vi "参数设置页.vi"() -> ()   [LabVIEW 2016, in "斯坦道总磷总氮.lvlib"]
uses:
  <vilib>/Plasmionique/MB Master/MB_Master/MB_Master.lvclass
  <vilib>/ptbypt/NI_PtbyPt.lvlib
panel:
  in  "简易流程路径":path=path "data/流程.xml"
  out "数据刷新时间":string
  in  "通讯连接":bool
  out "MB table":enum32{"Serial", "TCP"}(tab)
  in  "请选择串口:":refnum<visa-resource-name>
  in  "IP":string="127.0.0.1"
  in  "PORT":string="1001"
  in  "通信方式选择":enum16{"串口", "TCP"}(ring)
  in  "盐度自动补偿：":bool
  out "盐度补偿值":dbl caption="盐度补偿值："
  in  "刷新":bool
  in  "测量模式":T1(ring)
  in  "参数下拉列表":u16(ring) items=["总磷"=1, "总氮"=2]
  in  "量程下拉列表":enum16{"低量程", "高量程"}(ring)
  in  "测试流程路径":path=path "data/流程.xml"
  in  "标样核查量程模式":enum16{"高量程", "低量程", "自动"}(ring) caption="标样核查量程模式："
  in  "加标回收量程模式":enum16{"高量程", "低量程", "自动"}(ring) caption="加标回收量程模式："
  in  "跨度核查量程模式":enum16{"高量程", "低量程", "自动"}(ring) caption="跨度核查量程模式："
  in  "零点核查量程模式":enum16{"高量程", "低量程", "自动"}(ring) caption="零点核查量程模式："
  in  "水样测试量程模式":enum16{"高量程", "低量程", "自动"}(ring) caption="水样测试量程模式："
  out "稀释度":dbl caption="稀释度："
  out "阈值（高->低）":dbl caption="阈值（高->低）："
  out "阈值（低->高）":dbl caption="阈值（低->高）："
  out "量程下限":dbl caption="量程下限："
  out "量程上限":dbl caption="量程上限："
  out "检出限":dbl caption="检出限："
  out "曲线截距":dbl caption="曲线截距：" format="%#.6f"
  out "曲线斜率":dbl caption="曲线斜率：" format="%#.6f"
  out "二次多项式系数":dbl caption="二次多项式系数：" format="%#.6f"
  out "消解时长":dbl caption="消解时长："
  out "消解温度":dbl caption="消解温度："
  out "测量精度":u16 caption="测量精度："
  in  "标样核查标液浓度":dbl caption="标样核查标液浓度："
  in  "跨度核查标液浓度":dbl caption="跨度核查标液浓度："
  in  "零点核查标液浓度":dbl caption="零点核查标液浓度："
  in  "跨度值":dbl caption="跨度值："
  # "ppt"
  # "mg/L"
  # "mg/L"
  # "mg/L"
  # "mg/L"
  # "mg/L"
  # "min"
  # "℃"
  # "mg/L"
  # "mg/L"
  # "mg/L"
  # "mg/L"
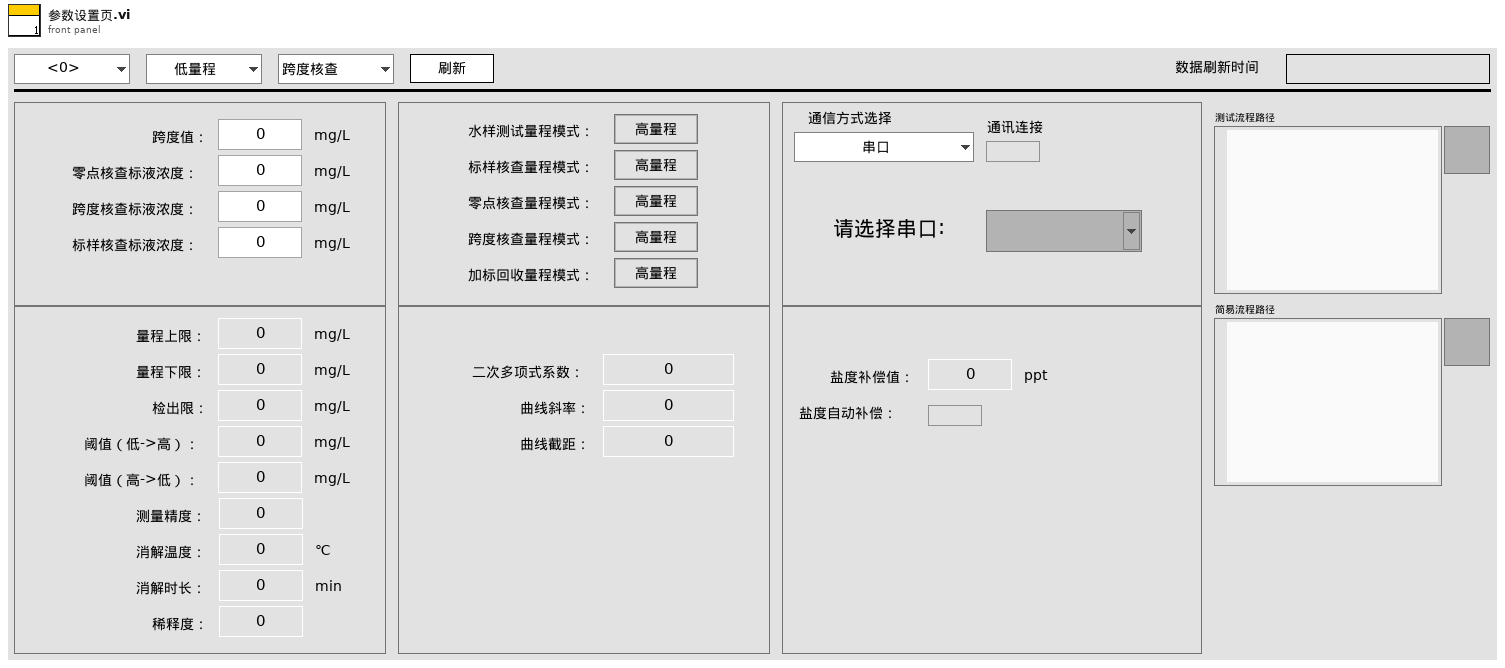
[diagram p1: front panel]
types:
  T1 = enum16{"跨度核查", "水样测量", "零点核查", "标样核查", "加标回收", "快捷测试", "空白校准", "标样校准"}
  T2 = enum8{"Enabled", "Disabled", "Disabled and Grayed Out"}
  T3 = typedef "LVStringsAndValuesArrayTypeDef_U16.ctl" = cluster{"String":string, "Value":u16}[]
  T4 = cluster{"标液浓度1":dbl, "测量吸光度1":dbl, "样品1启用":bool, "标液浓度2":dbl, "测量吸光度2":dbl, "样品2启用":bool, "标液浓度3":dbl, "测量吸光度3":dbl, "样品3启用":bool, "标液浓度4":dbl, "测量吸光度4":dbl, "样品4启用":bool, "标液浓度5":dbl, "测量吸光度5":dbl, "样品5启用":bool, "模型":enum32{"线性", "多项式"}, "精度":dbl, "XY图":cluster{"X Values":dbl[], "Y Values":dbl[]}[], "拟合公式":string, "r^2":dbl, "标样一校准时间":timestamp, "标样二校准时间":timestamp, "标样三校准时间":timestamp, "标样四校准时间":timestamp, "标样五校准时间":timestamp, "二次方程":cluster{"c":dbl, "x":dbl, "x^2":dbl}, "标定时间":timestamp}
  T5 = cluster{"系统时间":timestamp, "工作状态":u16, "测量模式":enum16{"待机", "连续模式", "周期模式", "定点模式", "受控模式", "手动模式"}, "告警代码":u16, "故障代码":u16, "日志代码":u16, "软件版本":u16, "F0":sgl, "F1":sgl, "F2":sgl, "F3":sgl, "T":sgl, "H":sgl, "id":u16, "flowid":u16, "量程":u16, "总磷控温温度1":sgl, "营养盐控温温度2":sgl, "ADC":sgl}
  T6 = cluster{"测量精度":u16, "检出限":dbl, "上限":dbl, "下限":dbl, "阈值（低->高）":dbl, "阈值（高->低）":dbl, "稀释度":dbl}
  T7 = cluster{"泵类型":u8, "进样速度":u32, "出样速度":u32, "泵阀量":u8, "光谱仪类型":u8, "光谱采样次数":u8, "氙灯次数":u8, "B":u16, "C":u16, "D":u16, "E":u16, "B_COD":u16, "C_COD":u16, "D_COD":u16, "E_COD":u16, "G":u16, "M":u16, "N":u16, "氨氮注射泵控温下限":sgl, "氨氮注射泵控温上限":sgl, "总氮注射泵控温下限":sgl, "总氮注射泵控温上限":sgl, "消解温度下限":sgl, "消解温度上限":sgl, "加热10s限值":sgl, "高温高压阀开阀温度":sgl, "总氮x公式0":u8, "总氮x公式1":sgl, "总氮x公式2":sgl, "总磷浊度稀释系数":sgl, "总磷浊度补偿权重1":sgl, "总磷浊度补偿权重2":sgl, "盐度系数":sgl, "氨氮补偿系数1":sgl, "氨氮补偿系数2":sgl}
  T8 = cluster{"标液浓度1":dbl, "测量吸光度1":dbl, "样品1启用":bool, "标液浓度2":dbl, "测量吸光度2":dbl, "样品2启用":bool, "标液浓度3":dbl, "测量吸光度3":dbl, "样品3启用":bool, "标液浓度4":dbl, "测量吸光度4":dbl, "样品4启用":bool, "标液浓度5":dbl, "测量吸光度5":dbl, "样品5启用":bool, "模型":enum32{"线性", "多项式"}, "精度":dbl, "XY图":cluster{"X Values":dbl[], "Y Values":dbl[]}[], "拟合公式":string, "r^2":dbl, "标样一校准时间":timestamp, "标样二校准时间":timestamp, "标样三校准时间":timestamp, "标样四校准时间":timestamp, "标样五校准时间":timestamp, "二次方程":cluster{"c":dbl, "x":dbl, "x^2":dbl}, "标定时间":timestamp}[]
  T9 = typedef "斯坦道总磷总氮.lvlib/关键参数.ctl" = cluster{"测量量程":sgl, "测量检出限":sgl, "测量精度":sgl, "测量间隔":sgl, "消解温度":sgl, "消解时长":sgl, "三项式系数":sgl, "二次多项式系数":sgl, "曲线斜率":sgl, "曲线截距":sgl, "线性相关系数":sgl, "空白校准时间":timestamp, "标样校准时间":timestamp, "测量信号值":sgl, "稀释倍数":sgl, "空白标定系数":sgl, "量程系数":sgl}
  T10 = cluster{"水样测试量程模式":enum16{"高量程", "低量程", "自动"}, "零点核查量程模式":enum16{"高量程", "低量程", "自动"}, "跨度核查量程模式":enum16{"高量程", "低量程", "自动"}, "加标回收量程模式":enum16{"高量程", "低量程", "自动"}, "标样核查量程模式":enum16{"高量程", "低量程", "自动"}}
  T11 = cluster{"总磷跨度值":dbl, "总磷零点标准液浓度":dbl, "总磷跨度标准液浓度":dbl, "总磷标准液标准浓度":dbl, "总氮跨度值":dbl, "总氮零点标准液浓度":dbl, "总氮跨度标准液浓度":dbl, "总氮标准液标准浓度":dbl, "COD跨度值":dbl, "COD零点标准液浓度":dbl, "COD跨度标准液浓度":dbl, "COD标准液标准浓度":dbl, "氨氮跨度值":dbl, "氨氮零点标准液浓度":dbl, "氨氮跨度标准液浓度":dbl, "氨氮标准液标准浓度":dbl, "磷酸盐跨度值":dbl, "磷酸盐零点标准液浓度":dbl, "磷酸盐跨度标准液浓度":dbl, "磷酸盐标准液标准浓度":dbl, "硝氮跨度值":dbl, "硝氮零点标准液浓度":dbl, "硝氮跨度标准液浓度":dbl, "硝氮标准液标准浓度":dbl, "亚硝氮跨度值":dbl, "亚硝氮零点标准液浓度":dbl, "亚硝氮跨度标准液浓度":dbl, "亚硝氮标准液标准浓度":dbl, "硫化物跨度值":dbl, "硫化物零点标准液浓度":dbl, "硫化物跨度标准液浓度":dbl, "硫化物标准液标准浓度":dbl, "硅酸盐跨度值":dbl, "硅酸盐零点标准液浓度":dbl, "硅酸盐跨度标准液浓度":dbl, "硅酸盐标准液标准浓度":dbl}
  T12 = cluster{"水样测试量程模式":u16, "零点核查量程模式":u16, "跨度核查量程模式":u16, "加标回收量程模式":u16, "标样核查量程模式":u16}
  T13 = cluster{"水样测试量程模式":enum16{"H", "L", "AUTO"}, "空白核查量程模式":enum16{"H", "L", "AUTO"}, "跨度核查量程模式":enum16{"H", "L", "AUTO"}, "加标回收量程模式":enum16{"H", "L", "AUTO"}, "标样核查量程模式":enum16{"H", "L", "AUTO"}}
  T14 = cluster{"水样测试量程模式":u16, "空白核查量程模式":u16, "跨度核查量程模式":u16, "加标回收量程模式":u16, "标样核查量程模式":u16}
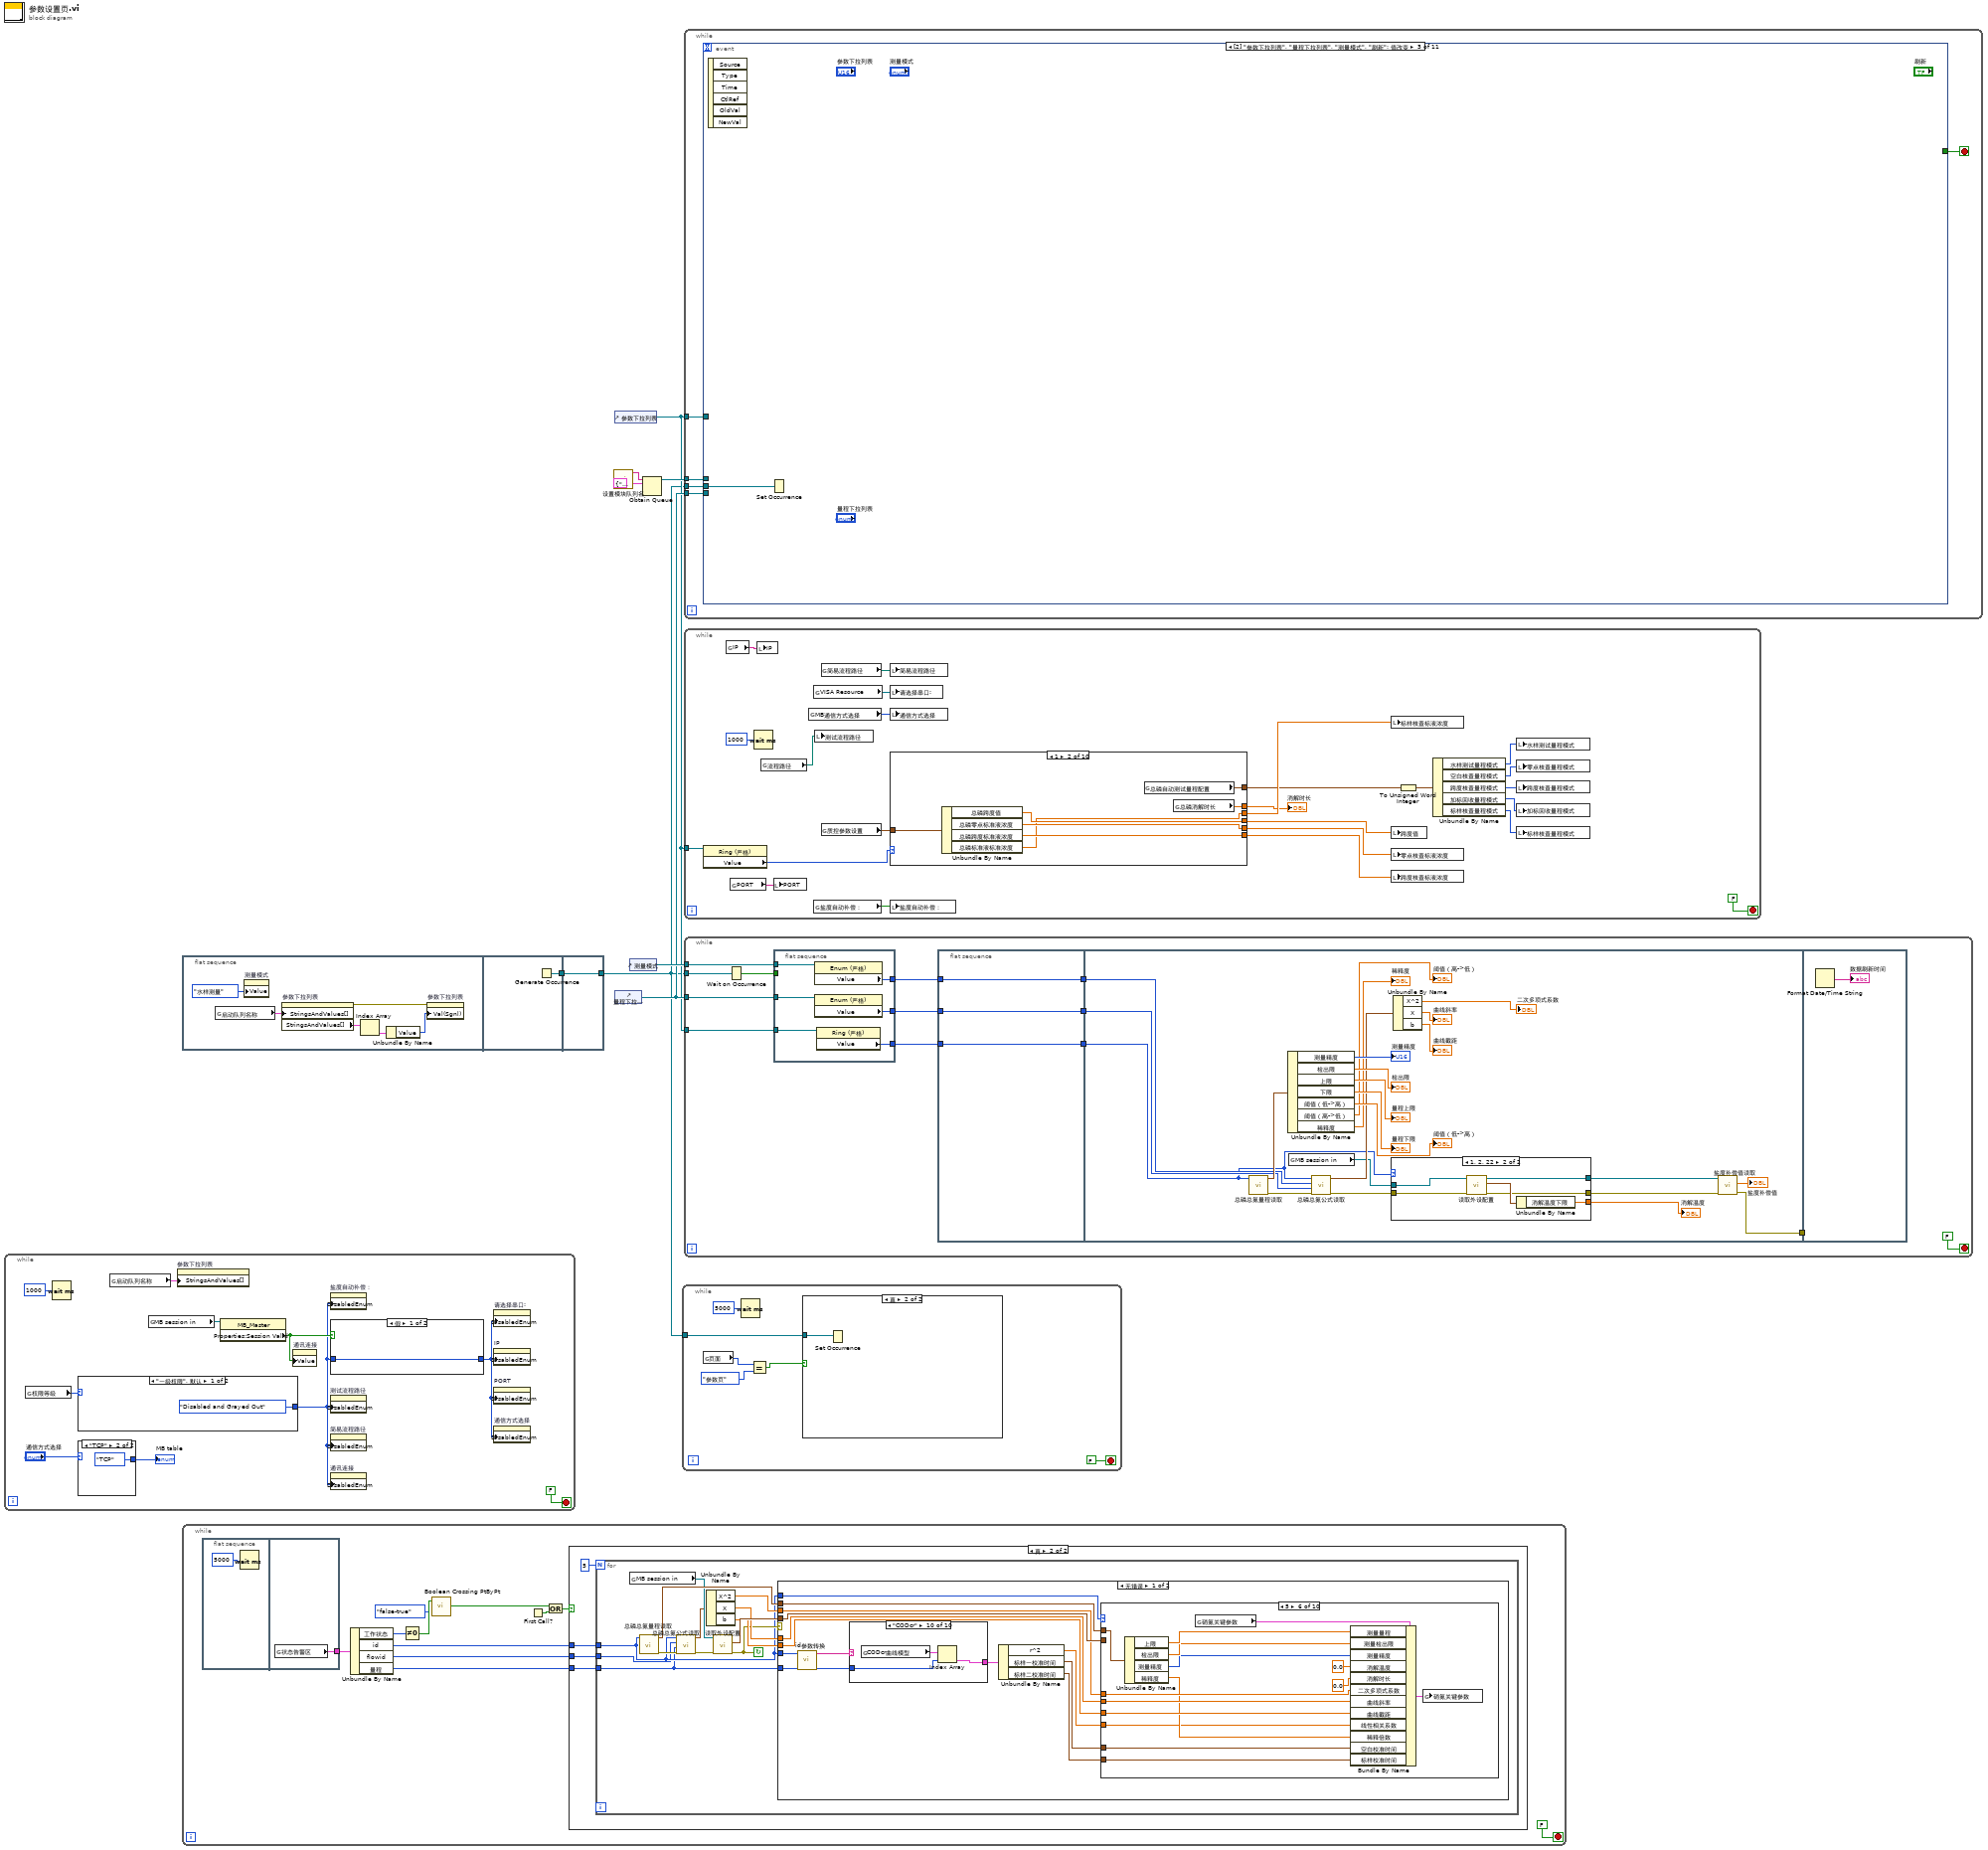
[diagram p0: block diagram]
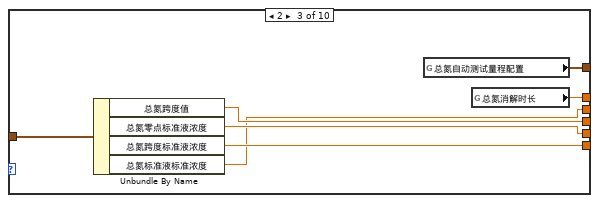
[diagram p4: hidden frame]
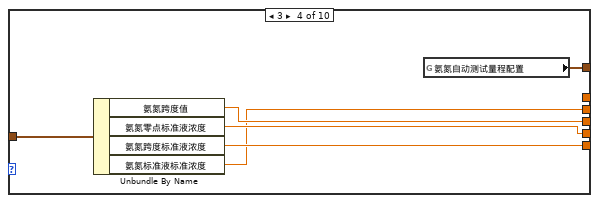
[diagram p5: hidden frame]
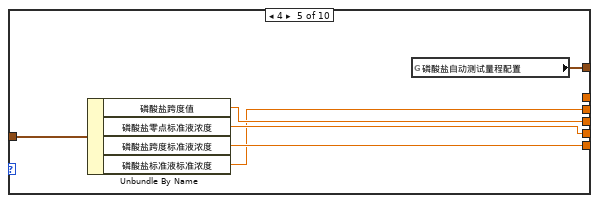
[diagram p6: hidden frame]
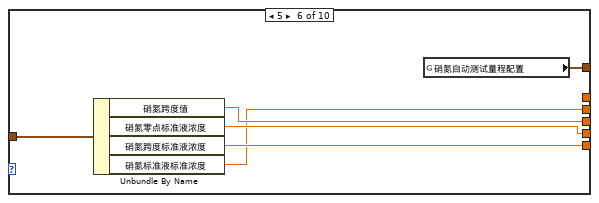
[diagram p7: hidden frame]
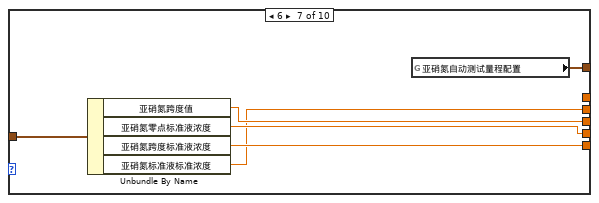
[diagram p8: hidden frame]
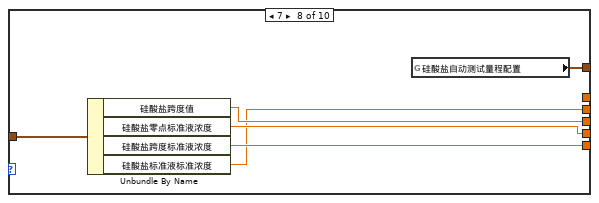
[diagram p9: hidden frame]
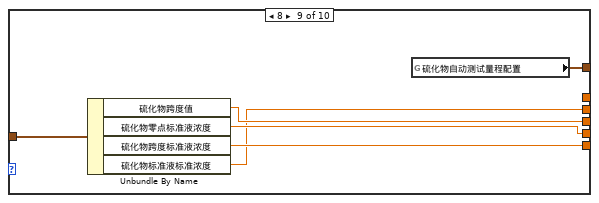
[diagram p10: hidden frame]
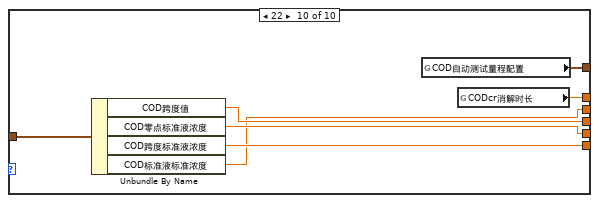
[diagram p11: hidden frame]
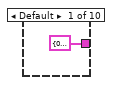
[diagram p13: hidden frame]
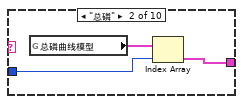
[diagram p14: hidden frame]
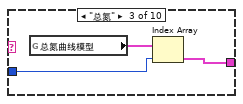
[diagram p15: hidden frame]
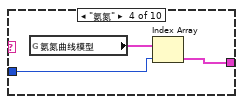
[diagram p16: hidden frame]
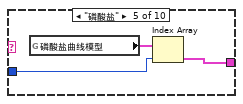
[diagram p17: hidden frame]
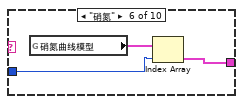
[diagram p18: hidden frame]
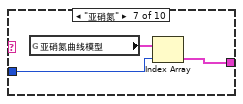
[diagram p19: hidden frame]
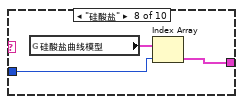
[diagram p20: hidden frame]
diagram:
  n1 = while {
    stop <- FALSE stop-if-true
    n2 = global read "VAR总磷总氮全局变量.vi" "权限等级"() -> (w11:enum16{"一级权限", "二级权限", "三级权限", "超级权限"})
    n3 = Wait (ms)(milliseconds to wait=u32 1000 ("等待时间（毫秒）")) -> ()  [unwired: 1 out]
    n4 = case shown="\"一级权限\", 默认" w11 {
      tunnel: [T2."Disabled and Grayed Out" ("禁用") T2."Enabled" ("禁用")] -> w10
      frame "一级权限", Default {
      }
      frame "二级权限".."超级权限" {
      }
    }
    n5 = case shown="\"TCP\"" "通信方式选择" {
      tunnel: [enum32{"Serial", "TCP"}."Serial" ("MB table") enum32{"Serial", "TCP"}."TCP" ("MB table")] -> w13
      frame "串口", Default {
      }
      frame "TCP" {
      }
    }
    "MB table" <- w13
    n6 = global read "总磷总氮断电保存全局变量.vi" "启动队列名称"() -> (w9:cluster{"String":string, "Value":u16}[])
    n7 = global read "VAR总磷总氮全局变量.vi" "MB session in"() -> (w17:refnum<class "MB_Master.lvclass">)
    n8 = property on="参数下拉列表" class="Ring (严格)"("StringsAndValues[]"=w9) -> ()  [unwired: 2 in, 2 out]
    n9 = property class="MB_Master"(reference=w17) -> ("Properties:Session Valid"=w15:bool)  [unwired: 1 in, 2 out]
    n10 = property on="通讯连接" class="Bool (严格)"("Value"=w15) -> ()  [unwired: 2 in, 2 out]
    n11 = property on="盐度自动补偿：" class="Bool (严格)"("DisabledEnum"=w10) -> ()  [unwired: 2 in, 2 out]
    n12 = case shown="假" w15 {
      tunnel: [w23 T2."Disabled and Grayed Out" ("禁用")] -> w14
      tunnel: w10 -> [w23 _]
      frame False {
      }
      frame True {
      }
    }
    n13 = property on="测试流程路径" class="Path"("DisabledEnum"=w10) -> ()  [unwired: 2 in, 2 out]
    n14 = property on="简易流程路径" class="Path"("DisabledEnum"=w10) -> ()  [unwired: 2 in, 2 out]
    n15 = property on="通讯连接" class="Bool (严格)"("DisabledEnum"=w10) -> ()  [unwired: 2 in, 2 out]
    n16 = property on="请选择串口:" class="VISAName"("DisabledEnum"=w14) -> ()  [unwired: 2 in, 2 out]
    n17 = property on="IP" class="Str"("DisabledEnum"=w14) -> ()  [unwired: 2 in, 2 out]
    n18 = property on="PORT" class="Str"("DisabledEnum"=w14) -> ()  [unwired: 2 in, 2 out]
    n19 = property on="通信方式选择" class="Enum (严格)"("DisabledEnum"=w14) -> ()  [unwired: 2 in, 2 out]
  }
  n20 = flat-sequence {
    tunnel: [w31] -> w8
    tunnel: [w32] -> w1
    tunnel: w8 -> [w32]
    frame #0 {
      n21 = global read "总磷总氮断电保存全局变量.vi" "启动队列名称"() -> (w26:cluster{"String":string, "Value":u16}[])
      n22 = property on="测量模式" class="Enum (严格)"("Value"=T1."水样测量" ("测量模式")) -> ()  [unwired: 2 in, 2 out]
      n23 = property on="参数下拉列表" class="Ring (严格)"("StringsAndValues[]"=w26) -> (error out=w29:errorcluster, "StringsAndValues[]"=w27:T3)  [unwired: 2 in, 1 out]
      n24 = Index Array(array=w27) -> (element=w28:cluster{"String":string, "Value":u16})  [unwired: 1 in]
      n25 = Unbundle By Name(w28) -> ("Value"=w30:u16)
      n26 = property on="参数下拉列表" class="Ring (严格)"(error in=w29, "Val(Sgnl)"=w30) -> ()  [unwired: 1 in, 2 out]
    }
    frame #1 {
      n27 = Generate Occurrence() -> (w31:refnum<k4>)
    }
    frame #2 {
    }
  }
  n28 = while {
    stop <- FALSE stop-if-true
    n29 = flat-sequence {
      tunnel: [w45] -> w43
      frame #0 {
        n30 = Wait (ms)(milliseconds to wait=u32 5000 ("等待时间（毫秒）")) -> ()  [unwired: 1 out]
      }
      frame #1 {
        n31 = global read "VAR总磷总氮全局变量.vi" "状态告警区"() -> (w45:T5)
      }
    }
    n32 = Unbundle By Name(w43) -> ("工作状态"=w39:u16, "id"=w40:u16, "flowid"=w41:u16, "量程"=w42:u16)
    n33 = Not Equal To 0?(x=w39) -> (x != 0?=w38:bool)
    n34 = call <vilib>:"Boolean Crossing PtByPt.vi"("direction"=enum16{"either", "false-true", "true-false"}."false-true", "input"=w38) -> ("crossing"=w36:bool)  [unwired: 1 in]
    n35 = First Call?() -> (First Call?: T/F=w33:bool)
    n36 = Or(x=w36, y=w33) -> (x .or. y?=w34:bool)
    n37 = case shown="真" w34 {
      tunnel: w42 -> [_ w49]
      tunnel: w41 -> [_ w48]
      tunnel: w40 -> [_ w47]
      frame False {
      }
      frame True {
        n38 = for {
          N: 5 -> [_]
          tunnel: w49 -> [w51]
          tunnel: w48 -> [w50]
          tunnel: w47 -> [w52]
          stop <- w53 continue-if-true
          n39 = global read "VAR总磷总氮全局变量.vi" "MB session in"() -> (w61:refnum<class "MB_Master.lvclass">)
          n40 = call "总磷总氮量程读取.vi"("测量参数"=w52) -> ("error out"=w55:errorcluster, "量程参数读取"=w62:T6)  [unwired: 9 in]
          n41 = call "总磷总氮公式读取.vi"("error in (no error)"=w55, "量程"=w51, "测量模式"=w50, "测量参数"=w52) -> ("error out"=w54:errorcluster, "公式"=w59:cluster{"X^2":dbl, "X":dbl, "b":dbl})  [unwired: 6 in]
          n42 = Unbundle By Name(w59) -> ("X^2"=w58:dbl, "X"=w57:dbl, "b"=w56:dbl)
          n43 = call "读取外设配置.vi"("error in (no error)"=w54, "MB session in"=w61) -> ("error out"=w53:errorcluster, "外设配置"=w60:T7)  [unwired: 7 in, 1 out]
          n44 = case shown="无错误" w53 {
            tunnel: w62 -> [w75 _]
            tunnel: w60 -> [w74 _]
            tunnel: w58 -> [w73 _]
            tunnel: w57 -> [w72 _]
            tunnel: w56 -> [w71 _]
            tunnel: w52 -> [w70 _]
            tunnel: w52 -> [w67 _]
            tunnel: w51 -> [w63 _]
            frame No Error {
              n45 = call "id参数转换.vi"("id"=w67) -> ("table输出"=w69:string)  [unwired: 9 in, 1 out]
              n46 = case shown="\"CODcr\"" w69 {
                tunnel: w63 -> [_ w77 w80 w83 w86 w89 w92 w95 w98 w101]
                tunnel: [T4 {"标液浓度1"=0.0, "测量吸光度1"=0.0, "样品1启用"=FALSE, "标液浓度2"=0.0, "测量吸光度2"=0.0, "样品2启用"=FALSE, "标液浓度3"=0.0, "测量吸光度3"=0.0, "样品3启用"=FALSE, "标液浓度4"=0.0, "测量吸光度4"=0.0, "样品4启用"=FALSE, "标液浓度5"=0.0, "测量吸光度5"=0.0, "样品5启用"=FALSE, "模型"=enum."线性", "精度"=0.0, "XY图"=[], "拟合公式"="", "r^2"=0.0, "标样一校准时间"=timestamp(0 s since 1904-01-01), "标样二校准时间"=timestamp(0 s since 1904-01-01), "标样三校准时间"=timestamp(0 s since 1904-01-01), "标样四校准时间"=timestamp(0 s since 1904-01-01), "标样五校准时间"=timestamp(0 s since 1904-01-01), "二次方程"={"c"=0.0, "x"=0.0, "x^2"=0.0}, "标定时间"=timestamp(0 s since 1904-01-01)} ("总磷曲线模型") w78 w81 w84 w87 w90 w93 w96 w99 w102] -> w68
                frame Default {
                }
                frame "总磷" {
                  n47 = global read "校准数据全局变量.vi" "总磷曲线模型"() -> (w79:T8)
                  n48 = Index Array(array=w79, index=w77) -> (element=w78:T4)
                }
                frame "总氮" {
                  n49 = global read "校准数据全局变量.vi" "总氮曲线模型"() -> (w82:T8)
                  n50 = Index Array(array=w82, index=w80) -> (element=w81:T4)
                }
                frame "氨氮" {
                  n51 = global read "校准数据全局变量.vi" "氨氮曲线模型"() -> (w85:T8)
                  n52 = Index Array(array=w85, index=w83) -> (element=w84:T4)
                }
                frame "磷酸盐" {
                  n53 = global read "校准数据全局变量.vi" "磷酸盐曲线模型"() -> (w88:T8)
                  n54 = Index Array(array=w88, index=w86) -> (element=w87:T4)
                }
                frame "硝氮" {
                  n55 = global read "校准数据全局变量.vi" "硝氮曲线模型"() -> (w91:T8)
                  n56 = Index Array(array=w91, index=w89) -> (element=w90:T4)
                }
                frame "亚硝氮" {
                  n57 = global read "校准数据全局变量.vi" "亚硝氮曲线模型"() -> (w94:T8)
                  n58 = Index Array(array=w94, index=w92) -> (element=w93:T4)
                }
                frame "硅酸盐" {
                  n59 = global read "校准数据全局变量.vi" "硅酸盐曲线模型"() -> (w97:T8)
                  n60 = Index Array(array=w97, index=w95) -> (element=w96:T4)
                }
                frame "硫化物" {
                  n61 = global read "校准数据全局变量.vi" "硫化物曲线模型"() -> (w100:T8)
                  n62 = Index Array(array=w100, index=w98) -> (element=w99:T4)
                }
                frame "CODcr" {
                  n63 = global read "校准数据全局变量.vi" "CODcr曲线模型"() -> (w103:T8)
                  n64 = Index Array(array=w103, index=w101) -> (element=w102:T4)
                }
              }
              n65 = Unbundle By Name(w68) -> ("r^2"=w66:dbl, "标样一校准时间"=w65:timestamp, "标样二校准时间"=w64:timestamp)
              n66 = case shown="5" w70 {
                tunnel: w75 -> [_ w117 w133 w148 w163 w178 w191 w206 w221 w237]
                tunnel: w74 -> [_ w113 w129 _ _ _ _ _ _ w229]
                tunnel: w73 -> [_ w110 w126 w144 w159 w174 w187 w202 w217 w233]
                tunnel: w72 -> [_ w109 w125 w143 w158 w173 w186 w201 w216 w232]
                tunnel: w71 -> [_ w108 w124 w142 w157 w172 w185 w200 w215 w231]
                tunnel: w66 -> [_ w104 w122 w138 w151 w168 _ w196 w209 w226]
                tunnel: w65 -> [_ w105 w121 w137 w153 w167 _ w195 w211 w225]
                tunnel: w64 -> [_ w106 w120 w136 w152 w166 _ w194 w210 w224]
                frame 0, Default {
                }
                frame 1 {
                  n67 = Unbundle By Name(w113) -> ("消解温度下限"=w112:sgl)
                  n68 = Unbundle By Name(w117) -> ("上限"=w116:dbl, "检出限"=w115:dbl, "测量精度"=w114:u16, "稀释度"=w107:dbl)
                  n69 = global read "VAR总磷总氮全局变量.vi" "总磷关键参数"() -> (w118:T9)
                  n70 = global read "总磷总氮断电保存全局变量.vi" "总磷消解时长"() -> (w111:dbl)
                  n71 = Bundle By Name(cluster=w118, "测量量程"=w116, "测量检出限"=w115, "测量精度"=w114, "消解温度"=w112, "消解时长"=w111, "二次多项式系数"=w110, "曲线斜率"=w109, "曲线截距"=w108, "线性相关系数"=w104, "稀释倍数"=w107, "空白校准时间"=w105, "标样校准时间"=w106) -> (w119:T9)
                  n72 = global write "VAR总磷总氮全局变量.vi" "总磷关键参数"(w119) -> ()
                }
                frame 2 {
                  n73 = Unbundle By Name(w129) -> ("消解温度下限"=w128:sgl)
                  n74 = Unbundle By Name(w133) -> ("上限"=w132:dbl, "检出限"=w131:dbl, "测量精度"=w130:u16, "稀释度"=w123:dbl)
                  n75 = global read "VAR总磷总氮全局变量.vi" "总氮关键参数"() -> (w134:T9)
                  n76 = global read "总磷总氮断电保存全局变量.vi" "总氮消解时长"() -> (w127:dbl)
                  n77 = Bundle By Name(cluster=w134, "测量量程"=w132, "测量检出限"=w131, "测量精度"=w130, "消解温度"=w128, "消解时长"=w127, "二次多项式系数"=w126, "曲线斜率"=w125, "曲线截距"=w124, "线性相关系数"=w122, "稀释倍数"=w123, "空白校准时间"=w121, "标样校准时间"=w120) -> (w135:T9)
                  n78 = global write "VAR总磷总氮全局变量.vi" "总氮关键参数"(w135) -> ()
                }
                frame 3 {
                  n79 = Unbundle By Name(w148) -> ("上限"=w147:dbl, "检出限"=w146:dbl, "测量精度"=w145:u16, "稀释度"=w141:dbl)
                  n80 = global read "VAR总磷总氮全局变量.vi" "氨氮关键参数"() -> (w149:T9)
                  n81 = Bundle By Name(cluster=w149, "测量量程"=w147, "测量检出限"=w146, "测量精度"=w145, "消解温度"=sgl 0.0, "消解时长"=sgl 0.0, "二次多项式系数"=w144, "曲线斜率"=w143, "曲线截距"=w142, "线性相关系数"=w138, "稀释倍数"=w141, "空白校准时间"=w137, "标样校准时间"=w136) -> (w150:T9)
                  n82 = global write "VAR总磷总氮全局变量.vi" "氨氮关键参数"(w150) -> ()
                }
                frame 4 {
                  n83 = Unbundle By Name(w163) -> ("上限"=w162:dbl, "检出限"=w161:dbl, "测量精度"=w160:u16, "稀释度"=w156:dbl)
                  n84 = global read "VAR总磷总氮全局变量.vi" "磷酸盐关键参数"() -> (w164:T9)
                  n85 = Bundle By Name(cluster=w164, "测量量程"=w162, "测量检出限"=w161, "测量精度"=w160, "消解温度"=sgl 0.0, "消解时长"=sgl 0.0, "二次多项式系数"=w159, "曲线斜率"=w158, "曲线截距"=w157, "线性相关系数"=w151, "稀释倍数"=w156, "空白校准时间"=w153, "标样校准时间"=w152) -> (w165:T9)
                  n86 = global write "VAR总磷总氮全局变量.vi" "磷酸盐关键参数"(w165) -> ()
                }
                frame 5 {
                  n87 = Unbundle By Name(w178) -> ("上限"=w177:dbl, "检出限"=w176:dbl, "测量精度"=w175:u16, "稀释度"=w171:dbl)
                  n88 = global read "VAR总磷总氮全局变量.vi" "硝氮关键参数"() -> (w179:T9)
                  n89 = Bundle By Name(cluster=w179, "测量量程"=w177, "测量检出限"=w176, "测量精度"=w175, "消解温度"=sgl 0.0, "消解时长"=sgl 0.0, "二次多项式系数"=w174, "曲线斜率"=w173, "曲线截距"=w172, "线性相关系数"=w168, "稀释倍数"=w171, "空白校准时间"=w167, "标样校准时间"=w166) -> (w180:T9)
                  n90 = global write "VAR总磷总氮全局变量.vi" "硝氮关键参数"(w180) -> ()
                }
                frame 6 {
                  n91 = Unbundle By Name(w191) -> ("上限"=w190:dbl, "检出限"=w189:dbl, "测量精度"=w188:u16, "稀释度"=w183:dbl)
                  n92 = global read "VAR总磷总氮全局变量.vi" "亚硝氮关键参数"() -> (w192:T9)
                  n93 = Bundle By Name(cluster=w192, "测量量程"=w190, "测量检出限"=w189, "测量精度"=w188, "消解温度"=sgl 0.0, "消解时长"=sgl 0.0, "二次多项式系数"=w187, "曲线斜率"=w186, "曲线截距"=w185, "线性相关系数"=sgl 1.0, "稀释倍数"=w183) -> (w193:T9)
                  n94 = global write "VAR总磷总氮全局变量.vi" "亚硝氮关键参数"(w193) -> ()
                }
                frame 7 {
                  n95 = Unbundle By Name(w206) -> ("上限"=w205:dbl, "检出限"=w204:dbl, "测量精度"=w203:u16, "稀释度"=w199:dbl)
                  n96 = global read "VAR总磷总氮全局变量.vi" "硅酸盐关键参数"() -> (w207:T9)
                  n97 = Bundle By Name(cluster=w207, "测量量程"=w205, "测量检出限"=w204, "测量精度"=w203, "消解温度"=sgl 0.0, "消解时长"=sgl 0.0, "二次多项式系数"=w202, "曲线斜率"=w201, "曲线截距"=w200, "线性相关系数"=w196, "稀释倍数"=w199, "空白校准时间"=w195, "标样校准时间"=w194) -> (w208:T9)
                  n98 = global write "VAR总磷总氮全局变量.vi" "硅酸盐关键参数"(w208) -> ()
                }
                frame 8 {
                  n99 = Unbundle By Name(w221) -> ("上限"=w220:dbl, "检出限"=w219:dbl, "测量精度"=w218:u16, "稀释度"=w214:dbl)
                  n100 = global read "VAR总磷总氮全局变量.vi" "硫化物关键参数"() -> (w222:T9)
                  n101 = Bundle By Name(cluster=w222, "测量量程"=w220, "测量检出限"=w219, "测量精度"=w218, "消解温度"=sgl 0.0, "消解时长"=sgl 0.0, "二次多项式系数"=w217, "曲线斜率"=w216, "曲线截距"=w215, "线性相关系数"=w209, "稀释倍数"=w214, "空白校准时间"=w211, "标样校准时间"=w210) -> (w223:T9)
                  n102 = global write "VAR总磷总氮全局变量.vi" "硫化物关键参数"(w223) -> ()
                }
                frame 22 {
                  n103 = Unbundle By Name(w229) -> ("消解温度下限"=w228:sgl)
                  n104 = Unbundle By Name(w237) -> ("上限"=w236:dbl, "检出限"=w235:dbl, "测量精度"=w234:u16, "稀释度"=w230:dbl)
                  n105 = global read "VAR总磷总氮全局变量.vi" "CODcr关键参数"() -> (w238:T9)
                  n106 = global read "总磷总氮断电保存全局变量.vi" "CODcr消解时长"() -> (w227:dbl)
                  n107 = Bundle By Name(cluster=w238, "测量量程"=w236, "测量检出限"=w235, "测量精度"=w234, "消解温度"=w228, "消解时长"=w227, "二次多项式系数"=w233, "曲线斜率"=w232, "曲线截距"=w231, "线性相关系数"=w226, "稀释倍数"=w230, "空白校准时间"=w225, "标样校准时间"=w224) -> (w239:T9)
                  n108 = global write "VAR总磷总氮全局变量.vi" "CODcr关键参数"(w239) -> ()
                }
              }
            }
            frame Error {
            }
          }
        }
      }
    }
  }
  n109 = call "设置模块队列名.vi"() -> ("Msg"=w6:string)  [unwired: 5 in]
  n110 = control-ref of="参数下拉列表"() -> (w2:refnum<vi>)
  n111 = control-ref of="量程下拉列表"() -> (w3:refnum<vi>)
  n112 = control-ref of="测量模式"() -> (w4:refnum<vi>)
  n113 = Obtain Queue(name (unnamed)=w6, element data type=cluster{"命令":string, "data":variant} {"命令"="", "data"=variant}) -> (queue out=w5:refnum<queue>)  [unwired: 3 in, 2 out]
  n114 = while {
    tunnel: w1 -> [w242]
    stop <- FALSE stop-if-true
    n115 = global read "VAR总磷总氮全局变量.vi" "页面"() -> (w244:enum16{"主页", "参数页", "校准页"})
    n116 = Wait (ms)(milliseconds to wait=u32 5000 ("等待时间（毫秒）")) -> ()  [unwired: 1 out]
    n117 = Equal?(x=w244, y=enum16{"主页", "参数页", "校准页"}."参数页" ("页面")) -> (x = y?=w243:bool)
    n118 = case shown="真" w243 {
      tunnel: w242 -> [_ w246]
      frame False {
      }
      frame True {
        n119 = Set Occurrence(w246) -> ()
      }
    }
  }
  n120 = while {
    tunnel: w1 -> [w250]
    tunnel: w2 -> [w249]
    tunnel: w5 -> [w248]
    tunnel: w3 -> [w247]
    stop <- w251 stop-if-true
    n121 = event shown="[2] \"参数下拉列表\", \"量程下拉列表\", \"测量模式\", \"刷新\": 值改变" {
      selector: _ -> [_ _ _ _ _ _ _ _ _ _ _]
      dyn-events: _ -> [_ _ _ _ _ _ _ _ _ _ _]
      timeout: _ -> [_ _ _ _ _ _ _ _ _ _ _]
      tunnel: [_ TRUE _ _ _ _ _ _ _ _ _] -> w251
      tunnel: w250 -> [_ _ w253 _ _ _ _ _ _ w300 _]
      tunnel: w249 -> [_ _ _ _ w272 _ _ _ _ w302 _]
      tunnel: w248 -> [_ _ _ _ _ _ _ _ _ _ w393]
      tunnel: w247 -> [_ _ _ _ _ _ _ _ _ _ _]
      event Timeout {
        n122 = event-data() -> ()  [unwired: 1 in, 3 out]
      }
      event Panel Close {
        n123 = event-data() -> ()  [unwired: 1 in, 4 out]
      }
      event "参数下拉列表", "量程下拉列表", "测量模式", "刷新": Value Change {
        n124 = event-data() -> ()  [unwired: 1 in, 6 out]
        n125 = Set Occurrence(w253) -> ()
      }
      event "跨度值", "零点核查标液浓度", "跨度核查标液浓度", "标样核查标液浓度", "消解温度", "消解时长", "检出限", "量程上限", "量程下限", "阈值（低->高）", "阈值（高->低）", "稀释度": Mouse Down {
        n126 = event-data() -> ("CtlRef"=w255:refnum<vi>)  [unwired: 1 in, 5 out]
        n127 = global read "VAR总磷总氮全局变量.vi" "权限等级"() -> (w254:enum16{"一级权限", "二级权限", "三级权限", "超级权限"})
        n128 = case shown="\"二级权限\"..\"超级权限\"" w254 {
          tunnel: w255 -> [_ w259]
          frame "一级权限", Default {
          }
          frame "二级权限".."超级权限" {
            n129 = property class="DigNum (严格)"(reference=w259) -> (reference out=w257:refnum<vi>, "Value"=w258:dbl)  [unwired: 1 in, 1 out]
            n130 = call "数字键盘.vi"("OldNumber"=w258) -> ("NewNumber"=w256:dbl)
            n131 = property class="DigNum (严格)"(reference=w257, "Val(Sgnl)"=w256) -> ()  [unwired: 1 in, 2 out]
          }
        }
      }
      event "测量精度", "检出限", "量程上限", "量程下限", "阈值（低->高）", "阈值（高->低）", "稀释度": Value Change {
        n132 = event-data() -> ()  [unwired: 1 in, 6 out]
        n133 = property class="Ring (严格)"(reference=w272) -> ("Value"=w271:u16)  [unwired: 1 in, 2 out]
        n134 = local read "阈值（低->高）"() -> (w265:dbl)
        n135 = local read "阈值（高->低）"() -> (w264:dbl)
        n136 = local read "测量精度"() -> (w262:u16)
        n137 = local read "量程上限"() -> (w268:dbl)
        n138 = local read "量程下限"() -> (w267:dbl)
        n139 = local read "检出限"() -> (w266:dbl)
        n140 = local read "稀释度"() -> (w263:dbl)
        n141 = Bundle By Name(cluster=T6 {"测量精度"=0, "检出限"=0.0, "上限"=0.0, "下限"=0.0, "阈值（低->高）"=0.0, "阈值（高->低）"=0.0, "稀释度"=0.0} ("量程参数写入"), "测量精度"=w262, "检出限"=w266, "上限"=w268, "下限"=w267, "阈值（低->高）"=w265, "阈值（高->低）"=w264, "稀释度"=w263) -> (w269:T6)
        n142 = call "总磷总氮量程写入.vi"("量程参数写入"=w269, "测量参数"=w271) -> ("error out"=w260:errorcluster)  [unwired: 8 in]
        n143 = case shown="错误" w260 {
          tunnel: ["写入成功" "写入失败"] -> w261
          frame No Error {
          }
          frame Error {
          }
        }
        n144 = One Button Dialog(message=w261) -> ()  [unwired: 1 in, 1 out]
      }
      event "消解温度": Value Change {
        n145 = event-data() -> ("NewVal"=w277:dbl)  [unwired: 1 in, 5 out]
        n146 = global read "VAR总磷总氮全局变量.vi" "MB session in"() -> (w278:refnum<class "MB_Master.lvclass">)
        n147 = call "读取外设配置.vi"("MB session in"=w278) -> ("error out"=w281:errorcluster, "外设配置"=w280:T7)  [unwired: 8 in, 1 out]
        n148 = Bundle By Name(cluster=w280, "消解温度下限"=w277) -> (w279:T7)
        n149 = call "写入外设配置.vi"("error in (no error)"=w281, "外设配置"=w279, "MB session in"=w278) -> ("error out"=w276:errorcluster)  [unwired: 7 in, 1 out]
        n150 = case shown="错误" w276 {
          tunnel: ["写入成功" "写入失败"] -> w275
          frame No Error {
          }
          frame Error {
          }
        }
        n151 = One Button Dialog(message=w275) -> ()  [unwired: 1 in, 1 out]
      }
      event "测量精度": Mouse Down {
        n152 = event-data() -> ("CtlRef"=w285:refnum<vi>)  [unwired: 1 in, 7 out]
        n153 = global read "VAR总磷总氮全局变量.vi" "权限等级"() -> (w284:enum16{"一级权限", "二级权限", "三级权限", "超级权限"})
        n154 = case shown="\"二级权限\"..\"超级权限\"" w284 {
          tunnel: w285 -> [_ w289]
          frame "一级权限", Default {
          }
          frame "二级权限".."超级权限" {
            n155 = property class="DigNum (严格)"(reference=w289) -> (reference out=w287:refnum<vi>, "Value"=w288:u16)  [unwired: 1 in, 1 out]
            n156 = call "数字键盘.vi"("OldNumber"=w288) -> ("NewNumber"=w286:dbl)
            n157 = property class="DigNum (严格)"(reference=w287, "Val(Sgnl)"=w286) -> ()  [unwired: 1 in, 2 out]
          }
        }
      }
      event "盐度补偿值": Mouse Down {
        n158 = event-data() -> ("CtlRef"=w291:refnum<vi>)  [unwired: 1 in, 3 out]
        n159 = global read "VAR总磷总氮全局变量.vi" "权限等级"() -> (w290:enum16{"一级权限", "二级权限", "三级权限", "超级权限"})
        n160 = case shown="\"二级权限\"..\"超级权限\"" w290 {
          tunnel: w291 -> [_ w293]
          frame "一级权限", Default {
          }
          frame "二级权限".."超级权限" {
            n161 = case shown="假" "盐度自动补偿：" {
              tunnel: w293 -> [w297 _]
              frame False {
                n162 = property class="DigNum (严格)"(reference=w297) -> (reference out=w295:refnum<vi>, "Value"=w296:dbl)  [unwired: 1 in, 1 out]
                n163 = call "数字键盘.vi"("OldNumber"=w296) -> ("NewNumber"=w294:dbl)
                n164 = property class="DigNum (严格)"(reference=w295, "Val(Sgnl)"=w294) -> ()  [unwired: 1 in, 2 out]
              }
              frame True {
              }
            }
          }
        }
      }
      event "盐度补偿值": Value Change {
        n165 = event-data() -> ("NewVal"=w298:dbl)  [unwired: 1 in, 5 out]
        n166 = global read "VAR总磷总氮全局变量.vi" "MB session in"() -> (w299:refnum<class "MB_Master.lvclass">)
        n167 = call "盐度补偿值写入.vi"("盐度补偿值"=w298, "MB session in"=w299) -> ()  [unwired: 8 in, 2 out]
      }
      event "跨度值", "零点核查标液浓度", "跨度核查标液浓度", "标样核查标液浓度", "消解时长", "水样测试量程模式", "零点核查量程模式", "跨度核查量程模式", "加标回收量程模式", "标样核查量程模式", "测试流程路径", "盐度自动补偿：", "IP", "PORT", "请选择串口:", "通信方式选择", "简易流程路径": Value Change {
        n168 = event-data() -> ()  [unwired: 1 in, 6 out]
        n169 = global read "VAR总磷总氮全局变量.vi" "权限等级"() -> (w301:enum16{"一级权限", "二级权限", "三级权限", "超级权限"})
        n170 = case shown="\"二级权限\"..\"超级权限\"" w301 {
          tunnel: w302 -> [_ w304]
          tunnel: w300 -> [w303 _]
          frame "一级权限", Default {
            n171 = Set Occurrence(w303) -> ()
          }
          frame "二级权限".."超级权限" {
            n172 = flat-sequence {
              tunnel: w304 -> [w325]
              frame #0 {
                n173 = property class="Ring (严格)"(reference=w325) -> ("Value"=w324:u16)  [unwired: 1 in, 2 out]
                n174 = global write "总磷总氮断电保存全局变量.vi" "PORT"("PORT") -> ()
                n175 = global write "总磷总氮断电保存全局变量.vi" "IP"("IP") -> ()
                n176 = local read "盐度自动补偿："() -> (w311:bool)
                n177 = local read "通信方式选择"() -> (w307:enum16{"串口", "TCP"})
                n178 = global write "总磷总氮断电保存全局变量.vi" "VISA Resource"("请选择串口:") -> ()
                n179 = global write "总磷总氮断电保存全局变量.vi" "简易流程路径"("简易流程路径") -> ()
                n180 = global write "总磷总氮断电保存全局变量.vi" "流程路径"("测试流程路径") -> ()
                n181 = global write "总磷总氮断电保存全局变量.vi" "MB通信方式选择"(w307) -> ()
                n182 = global write "总磷总氮断电保存全局变量.vi" "盐度自动补偿："(w311) -> ()
                n183 = Bundle("水样测试量程模式"="水样测试量程模式", "零点核查量程模式"="零点核查量程模式", "跨度核查量程模式"="跨度核查量程模式", "加标回收量程模式"="加标回收量程模式", "标样核查量程模式"="标样核查量程模式") -> (w313:T10)  [unwired: 1 in]
                n184 = global read "总磷总氮断电保存全局变量.vi" "质控参数设置"() -> (w319:T11)
                n185 = local read "消解时长"() -> (w306:dbl)
                n186 = To Unsigned Word Integer(number=w313) -> (unsigned 16bit integer=w312:T12)
                n187 = case shown="1" w324 {
                  tunnel: "跨度值" -> [_ w332 w340 w347 w354 w361 w368 w375 w382 w389]
                  tunnel: "标样核查标液浓度" -> [_ w329 w337 w344 w351 w358 w365 w372 w379 w386]
                  tunnel: "跨度核查标液浓度" -> [_ w330 w338 w345 w352 w359 w366 w373 w380 w387]
                  tunnel: "零点核查标液浓度" -> [_ w331 w339 w346 w353 w360 w367 w374 w381 w388]
                  tunnel: w319 -> [_ w334 w342 w349 w356 w363 w370 w377 w384 w391]
                  tunnel: w312 -> [_ w328 w336 w343 w350 w357 w364 w371 w378 _]
                  tunnel: w306 -> [_ w327 w335 _ _ _ _ _ _ w385]
                  frame 0, Default {
                  }
                  frame 1 {
                    n188 = global write "总磷总氮断电保存全局变量.vi" "总氮消解时长"(w327) -> ()
                    n189 = global write "总磷总氮断电保存全局变量.vi" "总磷自动测试量程配置"(w328) -> ()
                    n190 = Bundle By Name(cluster=w334, "总磷跨度值"=w332, "总磷零点标准液浓度"=w331, "总磷跨度标准液浓度"=w330, "总磷标准液标准浓度"=w329) -> (w333:T11)
                    n191 = global write "总磷总氮断电保存全局变量.vi" "质控参数设置"(w333) -> ()
                  }
                  frame 2 {
                    n192 = global write "总磷总氮断电保存全局变量.vi" "总氮消解时长"(w335) -> ()
                    n193 = global write "总磷总氮断电保存全局变量.vi" "总氮自动测试量程配置"(w336) -> ()
                    n194 = Bundle By Name(cluster=w342, "总氮跨度值"=w340, "总氮零点标准液浓度"=w339, "总氮跨度标准液浓度"=w338, "总氮标准液标准浓度"=w337) -> (w341:T11)
                    n195 = global write "总磷总氮断电保存全局变量.vi" "质控参数设置"(w341) -> ()
                  }
                  frame 3 {
                    n196 = global write "总磷总氮断电保存全局变量.vi" "氨氮自动测试量程配置"(w343) -> ()
                    n197 = Bundle By Name(cluster=w349, "氨氮跨度值"=w347, "氨氮零点标准液浓度"=w346, "氨氮跨度标准液浓度"=w345, "氨氮标准液标准浓度"=w344) -> (w348:T11)
                    n198 = global write "总磷总氮断电保存全局变量.vi" "质控参数设置"(w348) -> ()
                  }
                  frame 4 {
                    n199 = Bundle By Name(cluster=w356, "磷酸盐跨度值"=w354, "磷酸盐零点标准液浓度"=w353, "磷酸盐跨度标准液浓度"=w352, "磷酸盐标准液标准浓度"=w351) -> (w355:T11)
                    n200 = global write "总磷总氮断电保存全局变量.vi" "磷酸盐自动测试量程配置"(w350) -> ()
                    n201 = global write "总磷总氮断电保存全局变量.vi" "质控参数设置"(w355) -> ()
                  }
                  frame 5 {
                    n202 = global write "总磷总氮断电保存全局变量.vi" "硝氮自动测试量程配置"(w357) -> ()
                    n203 = Bundle By Name(cluster=w363, "硝氮跨度值"=w361, "硝氮零点标准液浓度"=w360, "硝氮跨度标准液浓度"=w359, "硝氮标准液标准浓度"=w358) -> (w362:T11)
                    n204 = global write "总磷总氮断电保存全局变量.vi" "质控参数设置"(w362) -> ()
                  }
                  frame 6 {
                    n205 = Bundle By Name(cluster=w370, "亚硝氮跨度值"=w368, "亚硝氮零点标准液浓度"=w367, "亚硝氮跨度标准液浓度"=w366, "亚硝氮标准液标准浓度"=w365) -> (w369:T11)
                    n206 = global write "总磷总氮断电保存全局变量.vi" "亚硝氮自动测试量程配置"(w364) -> ()
                    n207 = global write "总磷总氮断电保存全局变量.vi" "质控参数设置"(w369) -> ()
                  }
                  frame 7 {
                    n208 = Bundle By Name(cluster=w377, "硅酸盐跨度值"=w375, "硅酸盐零点标准液浓度"=w374, "硅酸盐跨度标准液浓度"=w373, "硅酸盐标准液标准浓度"=w372) -> (w376:T11)
                    n209 = global write "总磷总氮断电保存全局变量.vi" "硅酸盐自动测试量程配置"(w371) -> ()
                    n210 = global write "总磷总氮断电保存全局变量.vi" "质控参数设置"(w376) -> ()
                  }
                  frame 8 {
                    n211 = Bundle By Name(cluster=w384, "硫化物跨度值"=w382, "硫化物零点标准液浓度"=w381, "硫化物跨度标准液浓度"=w380, "硫化物标准液标准浓度"=w379) -> (w383:T11)
                    n212 = global write "总磷总氮断电保存全局变量.vi" "硫化物自动测试量程配置"(w378) -> ()
                    n213 = global write "总磷总氮断电保存全局变量.vi" "质控参数设置"(w383) -> ()
                  }
                  frame 22 {
                    n214 = global write "总磷总氮断电保存全局变量.vi" "CODcr消解时长"(w385) -> ()
                    n215 = Bundle By Name(cluster=w391, "COD跨度值"=w389, "COD零点标准液浓度"=w388, "COD跨度标准液浓度"=w387, "COD标准液标准浓度"=w386) -> (w390:T11)
                    n216 = global write "总磷总氮断电保存全局变量.vi" "质控参数设置"(w390) -> ()
                  }
                }
              }
              frame #1 {
                n217 = call "配置写入.vi"() -> ()  [unwired: 11 in, 1 out]
              }
            }
          }
        }
      }
      event "通讯连接": Value Change {
        n218 = event-data() -> ("NewVal"=w392:bool)  [unwired: 1 in, 5 out]
        n219 = Flush Queue(queue=w393) -> (queue out=w394:refnum<queue>)  [unwired: 1 in, 2 out]
        n220 = case shown="假" w392 {
          tunnel: w394 -> [w395 w397]
          frame False {
            n221 = Enqueue Element(queue=w395, element=cluster{"命令":string, "data":variant} {"命令"="停用模块", "data"=variant} ("元素")) -> ()  [unwired: 2 in, 3 out]
          }
          frame True {
            n222 = Enqueue Element(queue=w397, element=cluster{"命令":string, "data":variant} {"命令"="启用模块", "data"=variant} ("元素")) -> ()  [unwired: 2 in, 3 out]
          }
        }
      }
    }
  }
  n223 = while {
    tunnel: w2 -> [w401]
    stop <- FALSE stop-if-true
    n224 = property class="Ring (严格)"(reference=w401) -> ("Value"=w400:u16)  [unwired: 1 in, 2 out]
    n225 = global read "总磷总氮断电保存全局变量.vi" "IP"() -> (w418:string)
    n226 = global read "总磷总氮断电保存全局变量.vi" "PORT"() -> (w419:string)
    n227 = Wait (ms)(milliseconds to wait=u32 1000 ("等待时间（毫秒）")) -> ()  [unwired: 1 out]
    n228 = local write "IP"(w418) -> ()
    n229 = global read "总磷总氮断电保存全局变量.vi" "流程路径"() -> (w417:path)
    n230 = local write "PORT"(w419) -> ()
    n231 = global read "总磷总氮断电保存全局变量.vi" "MB通信方式选择"() -> (w415:enum16{"串口", "TCP"})
    n232 = global read "总磷总氮断电保存全局变量.vi" "VISA Resource"() -> (w420:refnum<visa-resource-name>)
    n233 = global read "总磷总氮断电保存全局变量.vi" "盐度自动补偿："() -> (w416:bool)
    n234 = local write "测试流程路径"(w417) -> ()
    n235 = global read "总磷总氮断电保存全局变量.vi" "简易流程路径"() -> (w399:path)
    n236 = global read "总磷总氮断电保存全局变量.vi" "质控参数设置"() -> (w410:T11)
    n237 = local write "简易流程路径"(w399) -> ()
    n238 = local write "请选择串口:"(w420) -> ()
    n239 = local write "通信方式选择"(w415) -> ()
    n240 = case shown="1" w400 {
      tunnel: [_ w429 w436 w442 w448 w454 w460 w466 w472 w479] -> w408
      tunnel: [_ w428 w435 _ _ _ _ _ _ w478] -> w409
      tunnel: w410 -> [_ w427 w434 w441 w447 w453 w459 w465 w471 w477]
      tunnel: [_ w426 w433 w440 w446 w452 w458 w464 w470 w476] -> w411
      tunnel: [_ w425 w432 w439 w445 w451 w457 w463 w469 w475] -> w412
      tunnel: [_ w424 w431 w438 w444 w450 w456 w462 w468 w474] -> w413
      tunnel: [_ w423 w430 w437 w443 w449 w455 w461 w467 w473] -> w414
      frame Default {
      }
      frame 1 {
        n241 = Unbundle By Name(w427) -> ("总磷跨度值"=w426:dbl, "总磷零点标准液浓度"=w425:dbl, "总磷跨度标准液浓度"=w424:dbl, "总磷标准液标准浓度"=w423:dbl)
        n242 = global read "总磷总氮断电保存全局变量.vi" "总磷自动测试量程配置"() -> (w429:T13)
        n243 = global read "总磷总氮断电保存全局变量.vi" "总磷消解时长"() -> (w428:dbl)
      }
      frame 2 {
        n244 = Unbundle By Name(w434) -> ("总氮跨度值"=w433:dbl, "总氮零点标准液浓度"=w432:dbl, "总氮跨度标准液浓度"=w431:dbl, "总氮标准液标准浓度"=w430:dbl)
        n245 = global read "总磷总氮断电保存全局变量.vi" "总氮自动测试量程配置"() -> (w436:T13)
        n246 = global read "总磷总氮断电保存全局变量.vi" "总氮消解时长"() -> (w435:dbl)
      }
      frame 3 {
        n247 = Unbundle By Name(w441) -> ("氨氮跨度值"=w440:dbl, "氨氮零点标准液浓度"=w439:dbl, "氨氮跨度标准液浓度"=w438:dbl, "氨氮标准液标准浓度"=w437:dbl)
        n248 = global read "总磷总氮断电保存全局变量.vi" "氨氮自动测试量程配置"() -> (w442:T13)
      }
      frame 4 {
        n249 = Unbundle By Name(w447) -> ("磷酸盐跨度值"=w446:dbl, "磷酸盐零点标准液浓度"=w445:dbl, "磷酸盐跨度标准液浓度"=w444:dbl, "磷酸盐标准液标准浓度"=w443:dbl)
        n250 = global read "总磷总氮断电保存全局变量.vi" "磷酸盐自动测试量程配置"() -> (w448:T13)
      }
      frame 5 {
        n251 = Unbundle By Name(w453) -> ("硝氮跨度值"=w452:dbl, "硝氮零点标准液浓度"=w451:dbl, "硝氮跨度标准液浓度"=w450:dbl, "硝氮标准液标准浓度"=w449:dbl)
        n252 = global read "总磷总氮断电保存全局变量.vi" "硝氮自动测试量程配置"() -> (w454:T13)
      }
      frame 6 {
        n253 = Unbundle By Name(w459) -> ("亚硝氮跨度值"=w458:dbl, "亚硝氮零点标准液浓度"=w457:dbl, "亚硝氮跨度标准液浓度"=w456:dbl, "亚硝氮标准液标准浓度"=w455:dbl)
        n254 = global read "总磷总氮断电保存全局变量.vi" "亚硝氮自动测试量程配置"() -> (w460:T13)
      }
      frame 7 {
        n255 = Unbundle By Name(w465) -> ("硅酸盐跨度值"=w464:dbl, "硅酸盐零点标准液浓度"=w463:dbl, "硅酸盐跨度标准液浓度"=w462:dbl, "硅酸盐标准液标准浓度"=w461:dbl)
        n256 = global read "总磷总氮断电保存全局变量.vi" "硅酸盐自动测试量程配置"() -> (w466:T13)
      }
      frame 8 {
        n257 = Unbundle By Name(w471) -> ("硫化物跨度值"=w470:dbl, "硫化物零点标准液浓度"=w469:dbl, "硫化物跨度标准液浓度"=w468:dbl, "硫化物标准液标准浓度"=w467:dbl)
        n258 = global read "总磷总氮断电保存全局变量.vi" "硫化物自动测试量程配置"() -> (w472:T13)
      }
      frame 22 {
        n259 = Unbundle By Name(w477) -> ("COD跨度值"=w476:dbl, "COD零点标准液浓度"=w475:dbl, "COD跨度标准液浓度"=w474:dbl, "COD标准液标准浓度"=w473:dbl)
        n260 = global read "总磷总氮断电保存全局变量.vi" "COD自动测试量程配置"() -> (w479:T13)
        n261 = global read "总磷总氮断电保存全局变量.vi" "CODcr消解时长"() -> (w478:dbl)
      }
    }
    "消解时长" <- w409
    n262 = local write "盐度自动补偿："(w416) -> ()
    n263 = local write "标样核查标液浓度"(w414) -> ()
    n264 = local write "跨度值"(w411) -> ()
    n265 = local write "零点核查标液浓度"(w412) -> ()
    n266 = local write "跨度核查标液浓度"(w413) -> ()
    n267 = To Unsigned Word Integer(number=w408) -> (unsigned 16bit integer=w407:T14)
    n268 = Unbundle By Name(w407) -> ("水样测试量程模式"=w406:u16, "空白核查量程模式"=w404:u16, "跨度核查量程模式"=w403:u16, "加标回收量程模式"=w402:u16, "标样核查量程模式"=w405:u16)
    n269 = local write "水样测试量程模式"(w406) -> ()
    n270 = local write "零点核查量程模式"(w404) -> ()
    n271 = local write "跨度核查量程模式"(w403) -> ()
    n272 = local write "加标回收量程模式"(w402) -> ()
    n273 = local write "标样核查量程模式"(w405) -> ()
  }
  n274 = while {
    tunnel: w2 -> [w491]
    tunnel: w3 -> [w490]
    tunnel: w4 -> [w489]
    tunnel: w1 -> [w488]
    stop <- FALSE stop-if-true
    n275 = Wait on Occurrence(2:w488) -> (0:w482:bool)  [unwired: 2 in]
    n276 = flat-sequence {
      tunnel: w491 -> [w498]
      tunnel: w490 -> [w497]
      tunnel: w489 -> [w496]
      tunnel: [w495] -> w485
      tunnel: [w494] -> w484
      tunnel: [w493] -> w483
      tunnel: w482 -> [_]
      frame #0 {
        n277 = property class="Enum (严格)"(reference=w496) -> ("Value"=w493:T1)  [unwired: 1 in, 2 out]
        n278 = property class="Enum (严格)"(reference=w497) -> ("Value"=w494:enum16{"低量程", "高量程"})  [unwired: 1 in, 2 out]
        n279 = property class="Ring (严格)"(reference=w498) -> ("Value"=w495:u16)  [unwired: 1 in, 2 out]
      }
    }
    n280 = flat-sequence {
      tunnel: [w501] -> w487
      tunnel: [w500] -> w486
      tunnel: w485 -> [w499]
      tunnel: w484 -> [w501]
      tunnel: w483 -> [w500]
      tunnel: [w499] -> w480
      tunnel: w487 -> [w510]
      tunnel: w486 -> [w511]
      tunnel: [w504] -> w481
      tunnel: w480 -> [w503]
      tunnel: w481 -> [_]
      frame #0 {
      }
      frame #1 {
        n281 = call "总磷总氮量程读取.vi"("测量参数"=w503) -> ("error out"=w516:errorcluster, "量程参数读取"=w524:T6)  [unwired: 9 in]
        n282 = Unbundle By Name(w524) -> ("测量精度"=→"测量精度":u16, "检出限"=→"检出限":dbl, "上限"=→"量程上限":dbl, "下限"=→"量程下限":dbl, "阈值（低->高）"=→"阈值（低->高）":dbl, "阈值（高->低）"=→"阈值（高->低）":dbl, "稀释度"=→"稀释度":dbl)
        n283 = global read "VAR总磷总氮全局变量.vi" "MB session in"() -> (w502:refnum<class "MB_Master.lvclass">)
        n284 = call "总磷总氮公式读取.vi"("error in (no error)"=w516, "量程"=w510, "测量模式"=w511, "测量参数"=w503) -> ("error out"=w505:errorcluster, "公式"=w515:cluster{"X^2":dbl, "X":dbl, "b":dbl})  [unwired: 6 in]
        n285 = case shown="1, 2, 22" w503 {
          tunnel: [w526 w532] -> w509
          tunnel: [_ w530] -> w508
          tunnel: [w525 w529] -> w507
          tunnel: w505 -> [w525 w528]
          tunnel: w502 -> [w526 w527]
          frame 0, Default {
          }
          frame 1, 2, 22 {
            n286 = call "读取外设配置.vi"("error in (no error)"=w528, "MB session in"=w527) -> ("error out"=w529:errorcluster, "外设配置"=w531:T7, "MB session out"=w532:refnum<class "MB_Master.lvclass">)  [unwired: 7 in]
            n287 = Unbundle By Name(w531) -> ("消解温度下限"=w530:sgl)
          }
        }
        "消解温度" <- w508
        n288 = Unbundle By Name(w515) -> ("X^2"=→"二次多项式系数":dbl, "X"=→"曲线斜率":dbl, "b"=→"曲线截距":dbl)
        n289 = call "盐度补偿值读取.vi"("Error in"=w507, "MB session in"=w509) -> ("error out"=w504:errorcluster, "盐度补偿值"=→"盐度补偿值":sgl)  [unwired: 7 in, 1 out]
      }
      frame #2 {
        n290 = Format Date/Time String() -> (date/time string=→"数据刷新时间":string)  [unwired: 3 in]
      }
    }
  }
